vi "LockIn.vi"() -> ()   [LabVIEW 2016]
uses:
  <vilib>/DAQmx/read.llb/DAQmx Read (Analog 1D Wfm NChan NSamp).vi
  <vilib>/DAQmx/create/channels.llb/DAQmx Create Channel (AI-Voltage-Basic).vi
  <vilib>/DAQmx/configure/timing.llb/DAQmx Timing (Sample Clock).vi
  <vilib>/DAQmx/miscellaneous.llb/DAQmx Fill In Error Info.vi
  <vilib>/Analysis/NI_AALPro.lvlib
panel:
  out "Amplitude History":dbl(graph)
  out "θ":dbl
  out "R":dbl
  out "Error Out":errorcluster caption="Error"
  in  "Stop":bool
  out "Y":dbl
  out "X":dbl
  out "# of elements in queue":i32
  in  "Allowance":dbl=0.1
  out "Measured Signal PLL'd":waveform(dbl)[](graph)=[{"t0"=timestamp(0 s since 1904-01-01), "dt"=2e-05, "Y"=array[5000 elements]}, {"t0"=timestamp(0.10000000000000002 s since 1904-01-01), "dt"=2e-05, "Y"=array[5000 elements]}]
  out "Measured Signal":waveform(dbl)[](graph)=[{"t0"=timestamp(0 s since 1904-01-01), "dt"=2e-05, "Y"=array[5000 elements]}, {"t0"=timestamp(0.10000000000000002 s since 1904-01-01), "dt"=2e-05, "Y"=array[5000 elements]}]
  in  "number of samples per channel":i32=5000
  in  "Maximum Value":dbl=10.0 format="%0.2f"
  in  "Minimum Value":dbl=-10.0 format="%0.2f"
  in  "Sample Rate":dbl=50000.0 caption="Sample Rate (Hz)" format="%0.2f"
  in  "Physical Channel":tag="cDAQ2Mod1/ai0:1"
  # "ai0 is for reference signal\nai1 is for signal went thorough DUT\nIf you don't have signal, please run\nAO Sample.vi before run this vi\nAO Sample\nao0 is for reference signal\nao1 is for signal went thorough DUT\nConnection Diagram. Tested by NI 9215 and NI 9263\nAI0+ ----- AO0\nAI0-  -----  COM\nAI1+ ----- AO1\nAI1-  ----- COM"
  # "Allowance means presicision of PLL\nPlease set this as positive value (>0)\nThe little the value is, the presicision will be good but\nit take more time to settle."
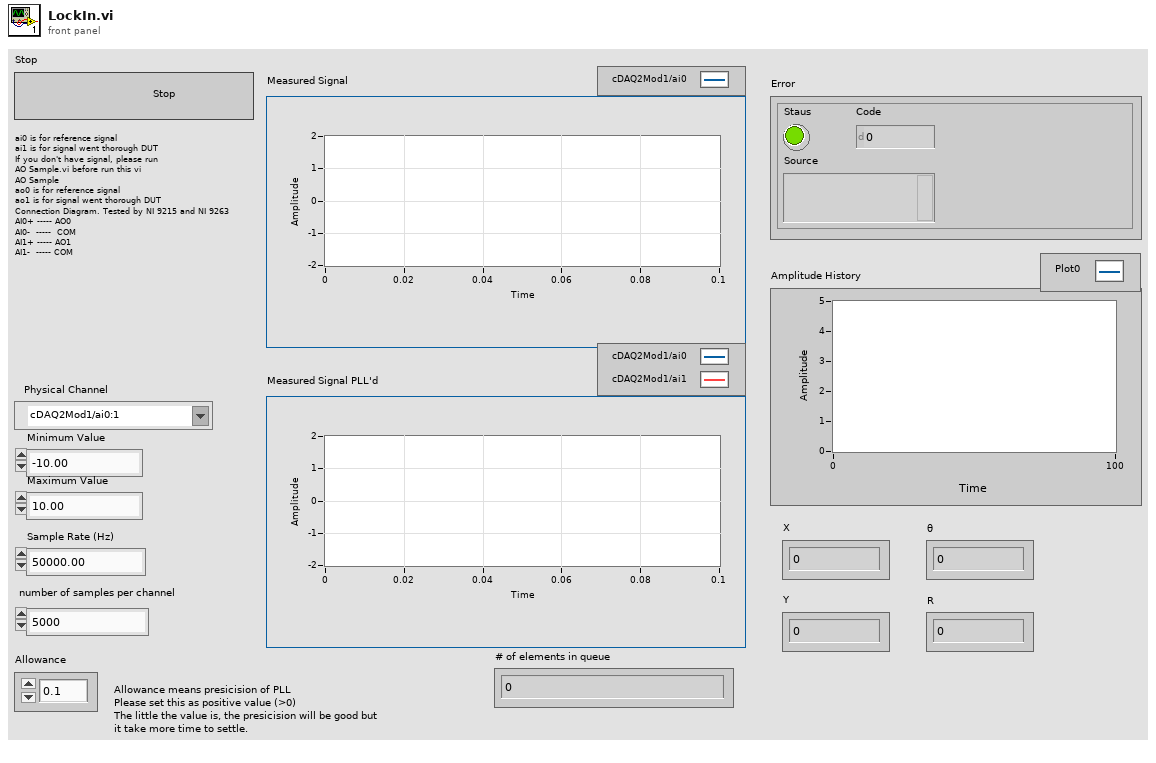
[diagram p1: front panel]
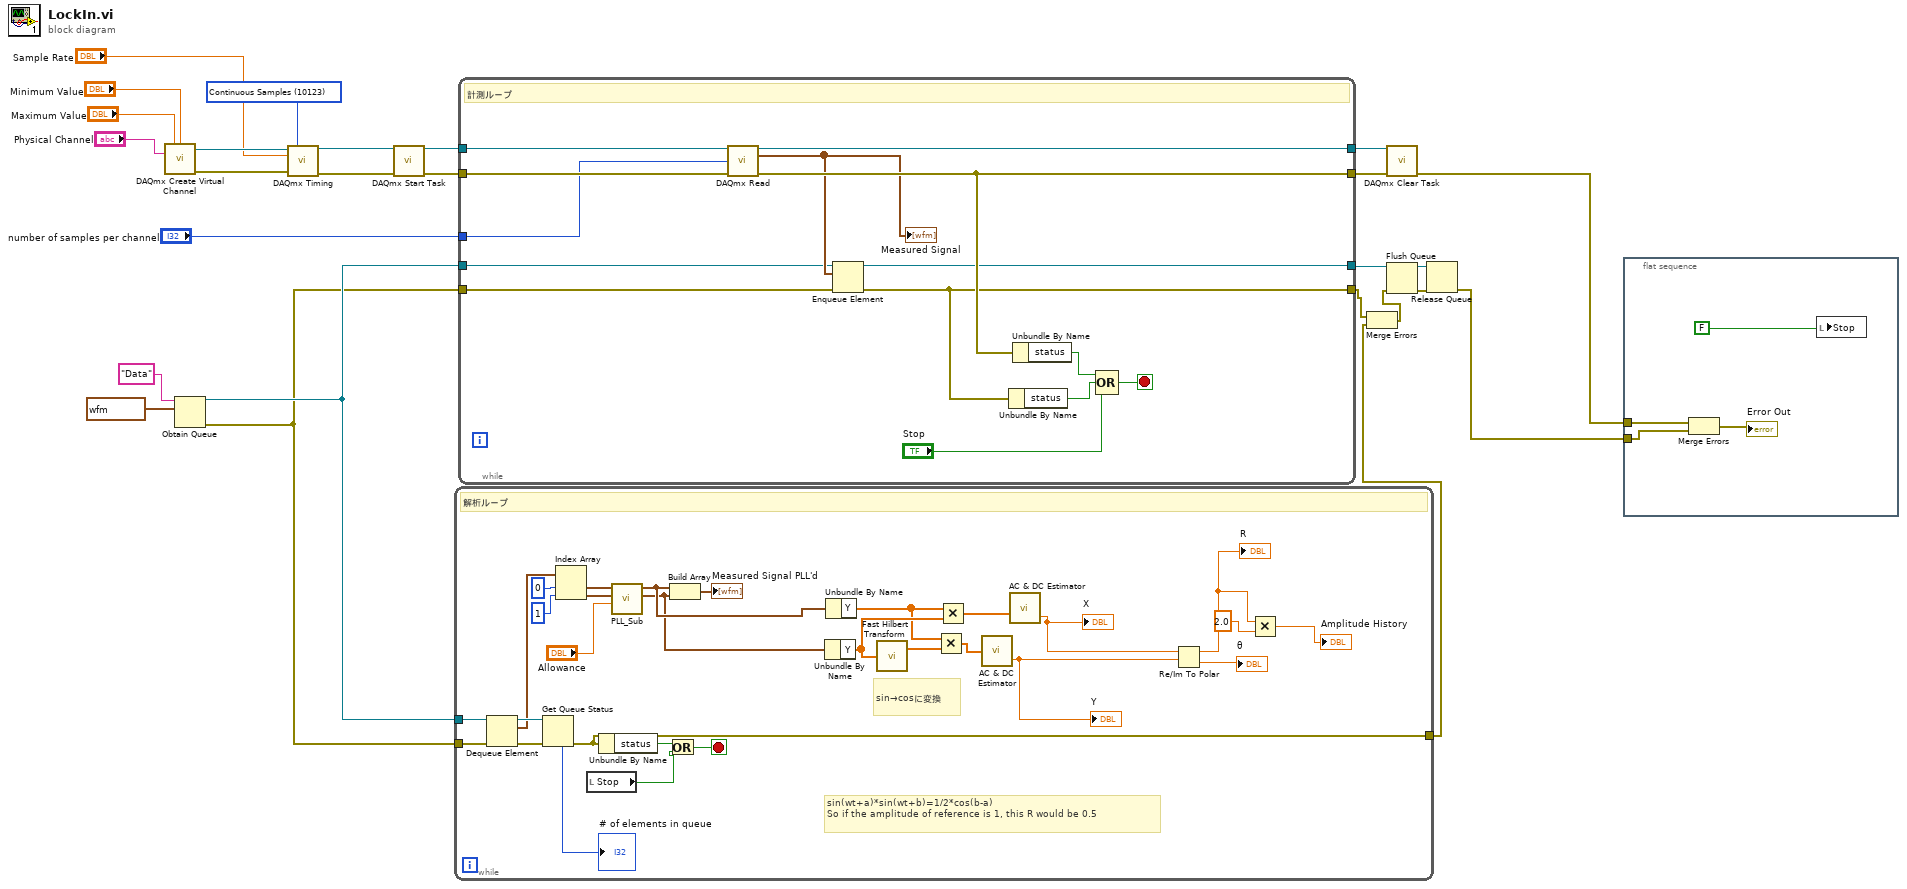
[diagram p0: block diagram]
diagram:
  w21 = 10123 items=["Finite Samples"=10178, "Continuous Samples"=10123] ("sample mode")
  n1 = call-poly <vilib>:"DAQmx Create Virtual Channel.vi"("maximum value"="Maximum Value", "minimum value"="Minimum Value", "physical channels"="Physical Channel") -> ("task out"=w23:refnum<k21>, "error out"=w24:errorcluster)  [unwired: 11 in]
  n2 = Obtain Queue(name (unnamed)="Data" ("名前（名前なし）"), element data type=waveform(dbl)[] [{"t0"=timestamp(3571029634.6453953 s since 1904-01-01), "dt"=1.9999999999999998e-05, "Y"=array[5000 elements]}, {"t0"=timestamp(3571029634.6453953 s since 1904-01-01), "dt"=1.9999999999999998e-05, "Y"=array[5000 elements]}] ("計測波形")) -> (queue out=w10:refnum<queue>, error out=w9:errorcluster)  [unwired: 3 in, 1 out]
  n3 = call-poly <vilib>:"DAQmx Timing.vi"("task/channels in"=w23, "sample mode"=w21, "rate"="Sample Rate", "error in"=w24) -> ("task out"=w20:refnum<k21>, "error out"=w19:errorcluster)  [unwired: 10 in]
  n4 = call <vilib>:"DAQmx Start Task.vi"("task/channels in"=w20, "error in"=w19) -> ("task out"=w17:refnum<k21>, "error out"=w18:errorcluster)  [unwired: 12 in]
  n5 = while {
    tunnel: w10 -> [w53]
    tunnel: w9 -> [w52]
    tunnel: [w42] -> w2
    stop <- w43 stop-if-true
    # "sin(wt+a)*sin(wt+b)=1/2*cos(b-a)\nSo if the amplitude of reference is 1, this R would be 0.5"
    # "sin→cosに変換"
    # "解析ループ"
    n6 = Dequeue Element(queue=w53, error in (no error)=w52) -> (queue out=w51:refnum<queue>, element=w49:waveform(dbl)[], error out=w50:errorcluster)  [unwired: 1 in, 1 out]
    n7 = Get Queue Status(queue=w51, error in (no error)=w50) -> (error out=w42:errorcluster, # elements in queue=→"# of elements in queue":i32)  [unwired: 1 in, 6 out]
    n8 = Index Array(array=w49, index #1=0 ("指標"), index #2=1 ("指標")) -> (element #1=w46:waveform(dbl), element #2=w45:waveform(dbl))
    n9 = local read "Stop"() -> (w33:bool)
    n10 = Unbundle By Name(w42) -> ("status"=w44:bool)
    n11 = call "PLL_Sub.vi"("Allowance"="Allowance", "Sig"=w45, "Ref"=w46) -> ("Sig Out Feed through"=w34:waveform(dbl), "Ref_PLL_Out"=w35:waveform(dbl))  [unwired: 7 in]
    n12 = Or(x=w44, y=w33) -> (x .or. y?=w43:bool)
    n13 = Build Array(w35, w34) -> (→"Measured Signal PLL'd":waveform(dbl)[])
    n14 = Unbundle By Name(w34) -> ("Y"=w39:dbl[])
    n15 = Unbundle By Name(w35) -> ("Y"=w38:dbl[])
    n16 = call <vilib>:"Fast Hilbert Transform.vi"("X"=w39) -> ("Hilbert{X}"=w40:dbl[])  [unwired: 1 out]
    n17 = Multiply(x=w38, y=w40) -> (x*y=w36:dbl[])
    n18 = Multiply(x=w38, y=w39) -> (x*y=w37:dbl[])
    n19 = call <vilib>:"AC & DC Estimator.vi"("Signal (V)"=w36) -> ("DC estimate (V)"=w31:dbl)  [unwired: 1 out]
    "Y" <- w31
    n20 = call <vilib>:"AC & DC Estimator.vi"("Signal (V)"=w37) -> ("DC estimate (V)"=w32:dbl)  [unwired: 1 out]
    "X" <- w32
    n21 = Re/Im To Polar(2:w31, 3:w32) -> (0:→"θ":dbl, 1:w29:dbl)
    "R" <- w29
    n22 = Multiply(x=w29, y=2.0) -> (x*y=→"Amplitude History":dbl)
  }
  n23 = while {
    tunnel: [w68] -> w16
    tunnel: [w69] -> w15
    tunnel: w18 -> [w67]
    tunnel: w17 -> [w66]
    tunnel: "number of samples per channel" -> [w65]
    tunnel: w10 -> [w63]
    tunnel: w9 -> [w62]
    tunnel: [w61] -> w6
    tunnel: [w60] -> w3
    stop <- w57 stop-if-true
    # "4."
    # "計測ループ"
    n24 = call-poly <vilib>:"DAQmx Read.vi"("task/channels in"=w66, "number of samples per channel"=w65, "error in"=w67) -> ("task out"=w68:refnum<k21>, "data"=w64:waveform(dbl)[], "error out"=w69:errorcluster)  [unwired: 10 in]
    "Measured Signal" <- w64
    n25 = Enqueue Element(queue=w63, element=w64, error in (no error)=w62) -> (queue out=w61:refnum<queue>, error out=w60:errorcluster)  [unwired: 1 in, 1 out]
    n26 = Unbundle By Name(w60) -> ("status"=w58:bool)
    n27 = Unbundle By Name(w69) -> ("status"=w59:bool)
    n28 = Compound Arithmetic op=OR ("複合演算")(w59, w58, "Stop") -> (w57:bool)
  }
  n29 = Merge Errors(w3, w2) -> (w1:errorcluster)
  n30 = call <vilib>:"DAQmx Clear Task.vi"("task in"=w16, "error in"=w15) -> ("error out"=w8:errorcluster)  [unwired: 13 in]
  n31 = Flush Queue(queue=w6, error in (no error)=w1) -> (queue out=w4:refnum<queue>, error out=w5:errorcluster)  [unwired: 1 out]
  n32 = Release Queue(queue=w4, error in (no error)=w5) -> (error out=w7:errorcluster)  [unwired: 1 in, 2 out]
  n33 = flat-sequence {
    tunnel: w8 -> [w73]
    tunnel: w7 -> [w70]
    frame #0 {
      n34 = Merge Errors(w73, w70) -> (→"Error Out":errorcluster)
      n35 = local write "Stop"(FALSE ("停止")) -> ()
    }
  }
